vi "LINX - PWM Set Duty Cycle Benchmark.vi"() -> ()   [LabVIEW 2014, in "LMH-LINX.lvlib"]
uses:
  vi.lib/MakerHub/LINX/Public/Peripherals/PWM/PWM Set Duty Cycle 1 Chan.vi
  vi.lib/MakerHub/LINX/Public/Utilities/Open Local.vi
  vi.lib/MakerHub/LINX/Public/Peripherals/PWM/PWM Set Duty Cycle N Chans.vi
  vi.lib/MakerHub/LINX/LMH-LINX.lvlib
panel:
  in  "Duty Cycle (0-1)":dbl=0.5
  in  "Warmup Iterations":i32=100
  out "Chart":dbl(graph)=10504.20168067227
  in  "Stop Button":bool
  in  "Benchmark Iterations":i32=1000
  out "Samples Per Second":i32
  in  "PWM Channel":u8=13
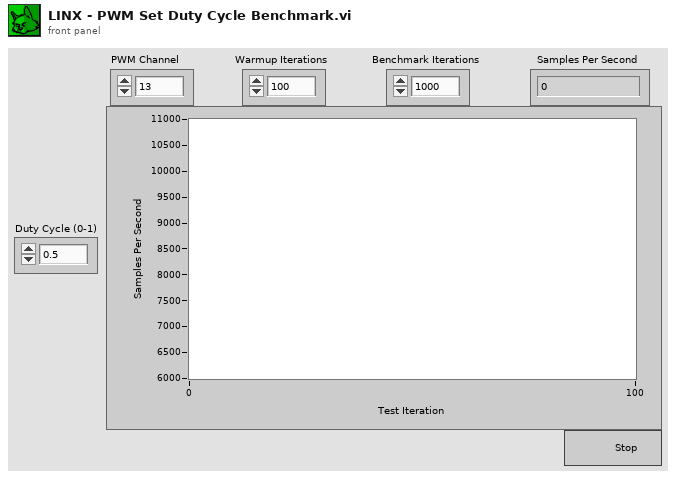
[diagram p1: front panel]
types:
  T1 = typedef "LMH-LINX.lvlib/LINX Ref.ctl" = cluster{"IO":T2, "Interface":T3, "LINX Device Config":T4}
  T2 = typedef "LMH-LINX.lvlib/Platform.ctl" = enum16{"Remote", "Local"}
  T3 = typedef "LMH-LINX.lvlib/Interface.ctl" = enum16{"Serial", "TCP"}
  T4 = typedef "LMH-LINX.lvlib/Device.lvlib/LINX Device Config.ctl" = cluster{"Interface":T3, "COM Port":refnum<visa-resource-name>, "TCP Configuration":T5, "Device Family":u8, "Device ID":u8, "Device Name":string, "TCP Ref":refnum<k5>, "Channels":T6}
  T5 = typedef "LMH-LINX.lvlib/Device.lvlib/TCP Config.ctl" = cluster{"IP Address":string, "Port":u16}
  T6 = typedef "LMH-LINX.lvlib/Channels.ctl" = cluster{"DI":u8[], "DO":u8[], "AI":u8[], "AO":u8[], "PWM":u8[], "QE":u8[], "UART":u8[], "I2C 2":u8[], "SPI":u8[], "CAN":u8[], "Servo":u8[], "AI Ref (V)":dbl, "AI Resolution (Bits)":u8, "AO Ref (V)":dbl, "AO Resolution (Bits)":u8}
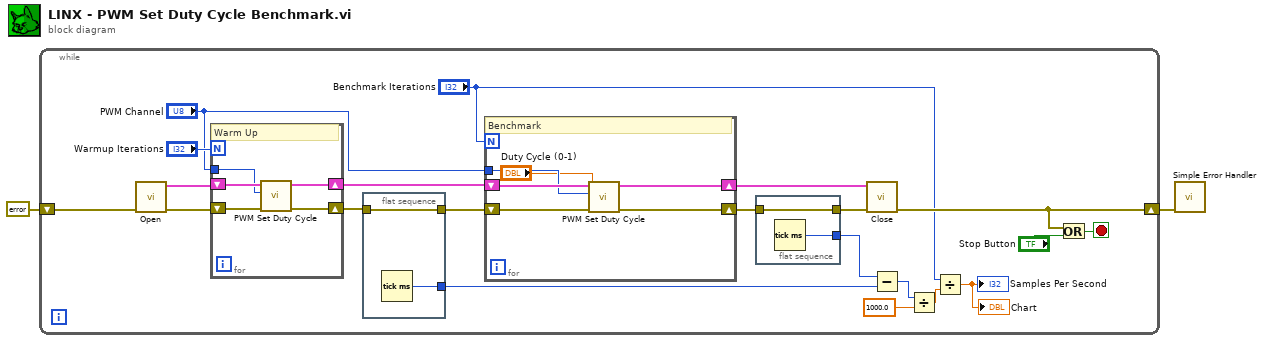
[diagram p0: block diagram]
diagram:
  n1 = while {
    shift-right: [w13] -> w2
    shift-left: errorcluster {"status"=FALSE, "code"=0, "source"=""} ("Error Out") -> [w11]
    stop <- w3 stop-if-true
    n2 = call-poly "Open.vi"("Error In"=w11) -> ("Error Out"=w18:errorcluster, "LINX Resource"=w19:T1)  [unwired: 8 in, 1 out]
    n3 = for {
      N: "Warmup Iterations" -> [_]
      shift-right: [w26] -> w16
      shift-left: w19 -> [w28]
      shift-right: [w25] -> w17
      shift-left: w18 -> [w27]
      tunnel: "PWM Channel" -> [w24]
      # "Warm Up"
      n4 = call-poly "PWM Set Duty Cycle.vi"("Error In"=w27, "PWM Channel"=w24, "LINX Resource"=w28) -> ("Error Out"=w25:errorcluster, "LINX Resource"=w26:T1)  [unwired: 7 in]
    }
    n5 = flat-sequence {
      tunnel: [w38] -> w22
      tunnel: w17 -> [w38]
      tunnel: [w37] -> w6
      frame #0 {
        n6 = Tick Count (ms)() -> (millisecond timer value=w37:u32)
      }
    }
    n7 = for {
      N: "Benchmark Iterations" -> [_]
      shift-right: [w32] -> w23
      shift-left: w16 -> [w34]
      shift-right: [w31] -> w21
      shift-left: w22 -> [w33]
      tunnel: "PWM Channel" -> [w30]
      # "Benchmark"
      n8 = call-poly "PWM Set Duty Cycle.vi"("Error In"=w33, "Duty Cycle (0-1)"="Duty Cycle (0-1)", "PWM Channel"=w30, "LINX Resource"=w34) -> ("Error Out"=w31:errorcluster, "LINX Resource"=w32:T1)  [unwired: 6 in]
    }
    n9 = flat-sequence {
      tunnel: [w36] -> w20
      tunnel: w21 -> [w36]
      tunnel: [w35] -> w7
      frame #0 {
        n10 = Tick Count (ms)() -> (millisecond timer value=w35:u32)
      }
    }
    n11 = call "Close.vi"("Error In"=w20, "LINX Resource"=w23) -> ("Error Out"=w13:errorcluster)  [unwired: 9 in]
    n12 = Subtract(x=w7, y=w6) -> (x-y=w10:u32)
    n13 = Divide(x=w10, y=1000.0) -> (x/y=w9:dbl)
    n14 = Divide(x="Benchmark Iterations", y=w9) -> (x/y=→"Chart" →"Samples Per Second":dbl)
    n15 = Or(x=w13, y="Stop Button") -> (x .or. y?=w3:bool)
  }
  n16 = call <vilib>:"Simple Error Handler.vi"("error in (no error)"=w2) -> ()  [unwired: 4 in, 5 out]
